vi "Handle Last Ack Core.vi"(4 "error in (no error)":errorcluster, 6 "Last Ack":refnum<class "Last Ack.lvclass">, 7 "Form Server in":refnum<class "Form Server.lvclass">) -> (0 "error out":errorcluster, 3 "Form Server out":refnum<class "Form Server.lvclass">)   [LabVIEW 2020, in "Form Server.lvlib" / "Form Server.lvclass"]
doc: "(<B>Filename</B>: Actor Framework.lvlib:Actor.lvclass:Handle Last Ack Core.vi)\n\nDefines how the caller actor responds to the Last Ack message from a nested actor. The Last Ack message is the final message a nested actor sends to its caller before it shuts down. The message contains information about the final state of the nested actor.\n\nBy default, this method does nothing except return any error the nested actor sent. A descendant class may override this method to define behavior."
uses:
  Form Server.lvclass
  <vilib>/ActorFramework/LastAck/Last Ack.lvclass
  <vilib>/ActorFramework/LastAck/Last Ack.lvclass/Last Ack.ctl
  Forms Model/Form Model Actor/Form Model.lvclass
  <vilib>/MGI/Monitored Actor/Monitored Actor/Monitored Actor/Monitored Actor.lvclass
  <vilib>/ActorFramework/Actor/Actor.lvclass
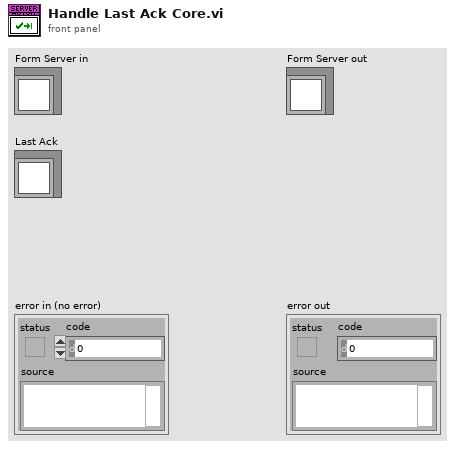
[diagram p1: front panel]
types:
  T1 = typedef "Form Server Interfaces.lvlib/Form ID.ctl" = cluster{"Name":string, "Panel type":string}
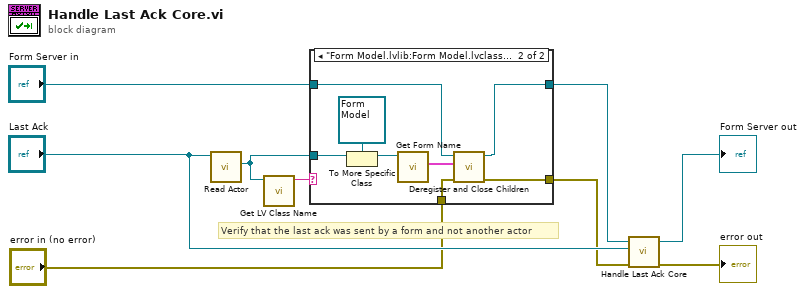
[diagram p0: block diagram]
diagram:
  # "Verify that the last ack was sent by a form and not another actor"
  n1 = call <vilib>:"Read Actor.vi"("Last Ack"="Last Ack") -> ("Actor"=w4:refnum<class "Actor.lvclass">)  [unwired: 10 in]
  n2 = call <vilib>:"Get LV Class Name.vi"("object"=w4) -> ("class name"=w2:string)  [unwired: 9 in, 1 out]
  n3 = case shown="\"Form Model.lvlib:Form Model.lvclass\"" w2 {
    tunnel: "Form Server in" -> [w11 w14]
    tunnel: [w11 w13] -> w5
    tunnel: w4 -> [_ w17]
    tunnel: "error in (no error)" -> [w10 w16]
    tunnel: [w10 w12] -> w3
    frame "", Default {
    }
    frame "Form Model.lvlib:Form Model.lvclass" {
      n4 = To More Specific Class(target class=refnum<class "Form Model.lvclass"> refnum ("Form Model.lvlib:Form Model.lvclass"), reference=w17) -> (specific class reference=w18:refnum<class "Form Model.lvclass">)  [unwired: 1 in, 1 out]
      n5 = call-dynamic "Get Form Name.vi"("Form Model in"=w18) -> ("Form ID"=w15:T1)  [unwired: 8 in, 2 out]
      n6 = call "Deregister and Close Children.vi"("error in (no error)"=w16, "Form Name"=w15, "Form Server in"=w14) -> ("error out"=w12:errorcluster, "Form Server out"=w13:refnum<class "Form Server.lvclass">)  [unwired: 7 in]
    }
  }
  n7 = call-parent "Handle Last Ack Core.vi"("error in (no error)"=w3, "Last Ack"="Last Ack", "Actor in"=w5) -> ("error out"=→"error out":errorcluster, "Actor out"=→"Form Server out":refnum<class "Form Server.lvclass">)  [unwired: 3 in]
